vi "Get Scanners.vi"(8 "error in (no error)":errorcluster, 11 "Double Scanner in":refnum<class "Double Scanner.lvclass">) -> (0 "error out":errorcluster, 1 "Scanner 2 out":refnum<class "Scanner.lvclass">, 2 "Scanner 1 out":refnum<class "Scanner.lvclass">, 3 "Double Scanner out":refnum<class "Double Scanner.lvclass">)   [LabVIEW 2017, in "Double Scanner.lvclass"]
uses:
  Double Scanner.lvclass
  Scanner/Scanner.lvclass
  Double Scanner.lvclass/Double Scanner.ctl
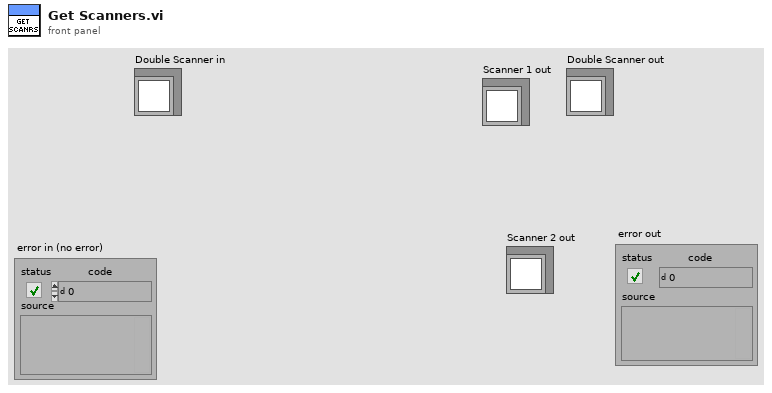
[diagram p1: front panel]
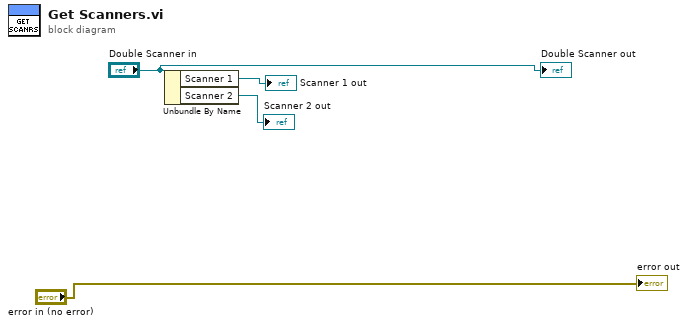
[diagram p0: block diagram]
diagram:
  n1 = Unbundle By Name("Double Scanner in") -> ("Scanner 1"=→"Scanner 1 out":refnum<class "Scanner.lvclass">, "Scanner 2"=→"Scanner 2 out":refnum<class "Scanner.lvclass">)
  "Double Scanner out" <- "Double Scanner in"
  "error out" <- "error in (no error)"
